vi "Add point in History v2.vi"(0 "History XY In":T2(array[cluster]), 1 "New Point":cluster{"X":dbl, "Y":dbl}, 3 "clear first (no:F)":bool, 4 "chart length (points)":i32=100) -> (5 "History XY Out":T1(array[cluster]))   [LabVIEW 2013]
panel:
  out "size(s)":i32
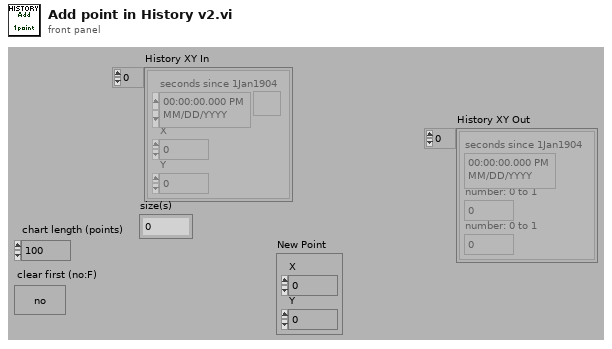
[diagram p1: front panel]
types:
  T1 = cluster{"seconds since 1Jan1904":timestamp, "number: 0 to 1":dbl, "number: 0 to 1":dbl}[]
  T2 = cluster{"seconds since 1Jan1904":timestamp, "X":dbl, "Y":dbl}[]
  T3 = cluster{"seconds since 1Jan1904":timestamp, "X":dbl, "Y":dbl}
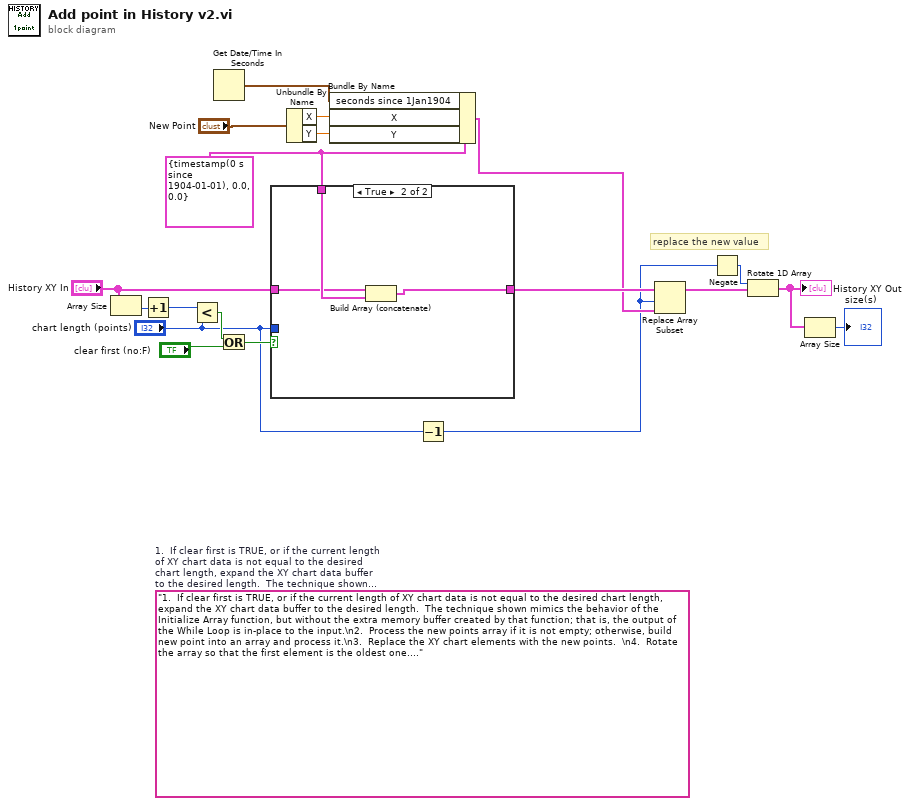
[diagram p0: block diagram]
diagram:
  w6 = T3 {"seconds since 1Jan1904"=timestamp(0 s since 1904-01-01), "X"=0.0, "Y"=0.0}
  (unwired) "1.  If clear first is TRUE, or if the current length of XY chart data is not equal to the desired chart length, expand the XY chart data buffer to the desired length.  The technique shown mimics the behavior of the Initialize Array function, but without the extra memory buffer created by that function; that is, the output of the While Loop is in-place to the input.\n2.  Process the new points array if it is not empty; otherwise, build new point into an array and process it.\n3.  Replace the XY chart elements with the new points.  \n4.  Rotate the array so that the first element is the oldest one.\nb marks a diagram array buffer; b? marks a buffer that may be in the calling VI. "  # 1.  If clear first is TRUE, or if the current length of XY chart data is not equal to the desired chart length, expand the XY chart data buffer to the desired length.  The technique shown mimics the behavior of the Initialize Array function, but without the extra memory buffer created by that function; that is, the output of the While Loop is in-place to the input. 2.  Process the new points array if it is not empty; otherwise, build new point into an array and process it. 3.  Replace the XY chart elements with the new points.   4.  Rotate the array so that the first element is the oldest one. b marks a diagram array buffer; b? marks a buffer that may be in the calling VI.
  # "replace the new value"
  n1 = Array Size(array="History XY In") -> (size(s)=w16:i32)
  n2 = Increment(x=w16) -> (x+1=w3:i32)
  n3 = Less?(x=w3, y="chart length (points)") -> (x < y?=w14:bool)
  n4 = Get Date/Time In Seconds() -> (seconds since 1Jan1904=w9:timestamp)
  n5 = Or(x=w14, y="clear first (no:F)") -> (x .or. y?=w13:bool)
  n6 = case shown="True" w13 {
    tunnel: [w20 w21] -> w17
    tunnel: "chart length (points)" -> [_ _]
    tunnel: "History XY In" -> [w20 w22]
    tunnel: w6 -> [_ w23]
    frame False {
    }
    frame True {
      n7 = Build Array (concatenate)(w22, w23) -> (w21:T2)
    }
  }
  n8 = Unbundle By Name("New Point") -> ("X"=w11:dbl, "Y"=w10:dbl)
  n9 = Bundle By Name(cluster=w6, "seconds since 1Jan1904"=w9, "X"=w11, "Y"=w10) -> (w7:T3)
  n10 = Decrement(x="chart length (points)") -> (x-1=w4:i32)
  n11 = Replace Array Subset(array=w17, new element=w7, index=w4) -> (w18:T2)
  n12 = Negate(x=w4) -> (-x=w19:i32)
  n13 = Rotate 1D Array(1:w18, 2:w19) -> (0:w2:T2)
  "History XY Out" <- w2
  n14 = Array Size(array=w2) -> (size(s)=→"size(s)":i32)
